vi "CANFD Stop.vi"(10 "CANIndex":u8, 11 "DevHandle":i32) -> (3 "function return":i32)   [LabVIEW 2010, in "usb2canfd.lvlib"]
doc: "int WINAPI CANFD_Stop(int DevHandle, unsigned char CANIndex);"
uses:
  usb2canfd.lvlib
  USB2XXX/trunk/USB2XXX/USB2XXX/vs2019/Release/USB2XXX.dll
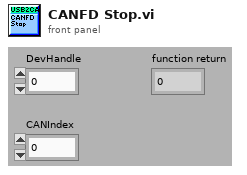
[diagram p1: front panel]
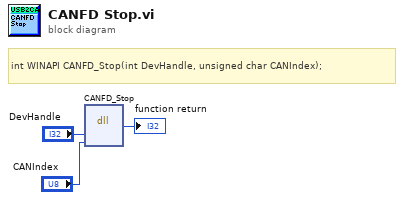
[diagram p0: block diagram]
diagram:
  # "int WINAPI CANFD_Stop(int DevHandle, unsigned char CANIndex);"
  n1 = dll-call lib="E:/Projects/USB2XXX/trunk/USB2XXX/USB2XXX/vs2019/Release/USB2XXX.*" fn="CANFD_Stop"("DevHandle"="DevHandle", "CANIndex"="CANIndex") -> (→"function return":i32)  [unwired: 5 in, 2 out]
